vi "card.vi"(4 "error in (no error)":errorcluster, 5 "count":u32) -> (0 "error out":errorcluster, 1 "comm_bus":u16, 2 "resource_name":string, 3 "status":i32)   [LabVIEW 8.6, in "ZTScopeM.lvlib"]
doc: "Returns all C-Class and M-Class ZTEC instruments. To find all cards increment count. While the return status is ZT_SUCCESS another card has been successfully found. A return of ZT_FAILURE indicated there are no more valid cards to be found."
uses:
  ZTScopeM.lvlib
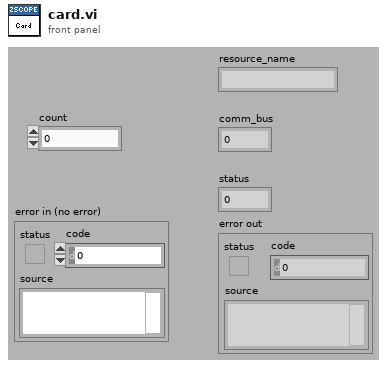
[diagram p1: front panel]
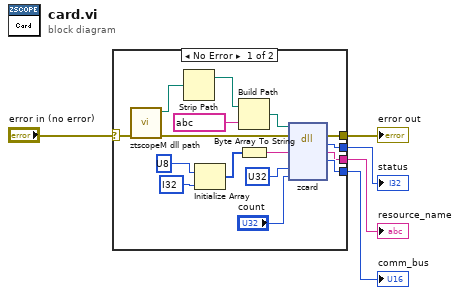
[diagram p0: block diagram]
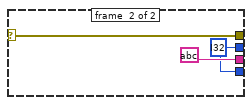
[diagram p2: hidden frame]
diagram:
  n1 = case shown="No Error" "error in (no error)" {
    selector: "error in (no error)" -> [w8 w24]
    tunnel: [w20 w22] -> w5
    tunnel: [w19 string ?] -> w4
    tunnel: [w13 w22] -> w3
    tunnel: [w6 w24] -> w1
    frame #0 {
      n2 = call "ztscopeM dll path.vi"("error in (no error)"=w8) -> ("error out"=w7:errorcluster, "<instrument>.dll path"=w10:path)  [unwired: 9 in]
      n3 = Strip Path(path=w10) -> (stripped path=w12:path)  [unwired: 1 out]
      n4 = Initialize Array(u8 ?, i32 ? ("dimension size")) -> (w16:u8[])
      n5 = Build Path(base path=w12, name or relative path=string ?) -> (appended path=w9:path)
      n6 = Byte Array To String(unsigned byte array=w16) -> (string=w14:string)
      n7 = dll-call lib="zcard.dll" fn="zcard"(path in=w9, error in=w7, "resource_name"=w14, "length"=u32 ?, "count"="count") -> (error out=w6:errorcluster, "return type"=w13:i32, "resource_name"=w19:string, "comm_bus"=w20:u16)  [unwired: 4 in, 1 out]
    }
    frame #1 {
      w22 = i32 ? ("return type")
    }
  }
  "resource_name" <- w4
  "comm_bus" <- w5
  "status" <- w3
  "error out" <- w1
